vi "ByteArrayToImage.vi"(0 "CameraBytes":u8[](array[numeric]), 1 "Image":T1) -> (5 "Image Out":T1)   [LabVIEW 2022 SP3]
uses:
  <vilib>/vision/NI_Vision_Development_Module.lvlib
  <vilib>/vision/Image Controls.llb/IMAQ Image.ctl
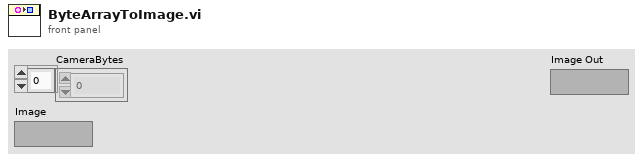
[diagram p1: front panel]
types:
  T1 = typedef "IMAQ Image.ctl" = refnum<image>
  T2 = cluster{"Red or Hue value":u8, "Green or Sat value":u8, "Blue or Luma or Val or Inten value":u8}
  T3 = cluster{"Red or Hue value":u8, "Green or Sat value":u8, "Blue or Luma or Val or Inten value":u8}[]
  T4 = cluster{"Red or Hue value":u8, "Green or Sat value":u8, "Blue or Luma or Val or Inten value":u8}[][]
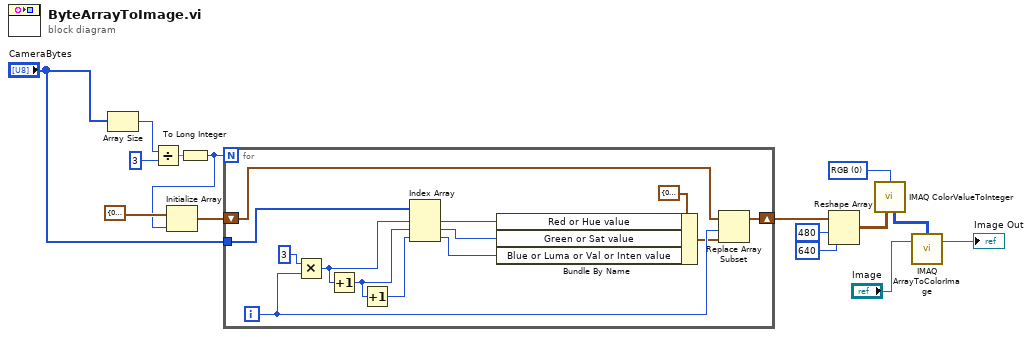
[diagram p0: block diagram]
diagram:
  w6 = u16 0 items=["RGB", "HSL", "HSV", "HSI"] ("Color Mode")
  n1 = Array Size(array="CameraBytes") -> (size(s)=w15:i32)
  n2 = Divide(x=w15, y=3) -> (x/y=w13:dbl)
  n3 = To Long Integer(number=w13) -> (32bit integer=w3:i32)
  n4 = Initialize Array(T2 {"Red or Hue value"=0, "Green or Sat value"=0, "Blue or Luma or Val or Inten value"=0} ("Color Value"), w3) -> (w11:T3)
  n5 = for {
    N: w3 -> [_]
    tunnel: "CameraBytes" -> [w26]
    shift-right: [w17] -> w10
    shift-left: w11 -> [w16]
    i -> [w19]
    n6 = Multiply(x=3, y=w19) -> (x*y=w22:i32)
    n7 = Increment(x=w22) -> (x+1=w21:i32)
    n8 = Increment(x=w21) -> (x+1=w20:i32)
    n9 = Index Array(array=w26, index #1=w22, index #2=w21, index #3=w20) -> (element #1=w25:u8, element #2=w24:u8, element #3=w23:u8)
    n10 = Bundle By Name(cluster=T2 {"Red or Hue value"=0, "Green or Sat value"=0, "Blue or Luma or Val or Inten value"=0} ("Color Value"), "Red or Hue value"=w25, "Green or Sat value"=w24, "Blue or Luma or Val or Inten value"=w23) -> (w18:T2)
    n11 = Replace Array Subset(array=w16, new element=w18, index=w19) -> (w17:T3)
  }
  n12 = Reshape Array(w10, 480 ("dimension size"), 640 ("dimension size")) -> (w7:T4)
  n13 = call "IMAQ ColorValueToInteger"("2D Color value array"=w7, "Color Mode"=w6) -> ("2D U32 array"=w5:u32[][])  [unwired: 3 in, 3 out]
  n14 = call "IMAQ ArrayToColorImage"("Image Pixels (U32)"=w5, "Image"="Image") -> ("Image Out"=→"Image Out":T1)  [unwired: 3 in, 1 out]
